vi "TOOLweb Zeit-Datum-Strings nach Zeitstempel.vi"(2 "Format":T1(ring), 3 "Zeit/Datum-String":string) -> (0 "Zeit-Cluster":T2, 1 "Zeitstempel":timestamp)   [LabVIEW 2020, in "FT-IR.lvlib" / "TOOLweb Interface.lvlib" / "TOOLweb Interface Hilfs-VIs.lvlib"]
doc: "Formt den TOOLweb-Zeit/Datum-String in einen Zeitstempel um. Der Ausgang \"Zeit-Cluster\" bietet einen einfachen Zugriff auf die einzelnen Elemente der Zeit/Datums-Information."
uses:
  TOOLweb Interface Hilfs-VIs.lvlib
  <vilib>/Utility/miscctls.llb/LVDateTimeRec.ctl
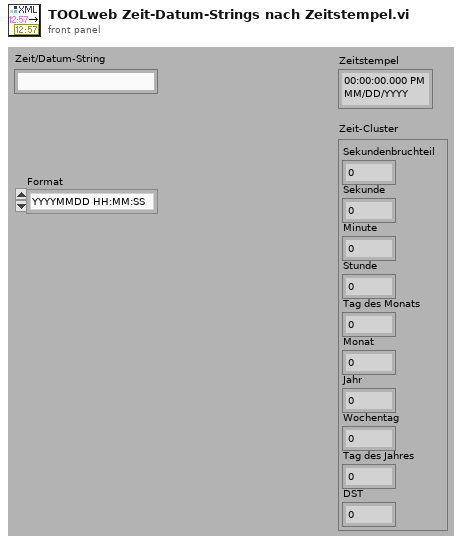
[diagram p1: front panel]
types:
  T1 = enum16{"YYYYMMDD HH:MM:SS", "[YYMMDD][HH:MM:SS]"}
  T2 = typedef "LVDateTimeRec.ctl" = cluster{"fractional second":dbl, "second":i32, "minute":i32, "hour":i32, "day of month":i32, "month":i32, "year":i32, "day of week":i32, "day of year":i32, "DST":i32}
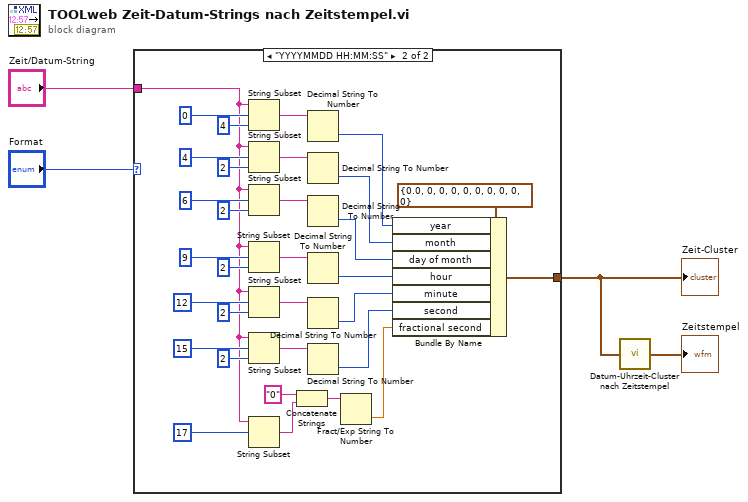
[diagram p0: block diagram]
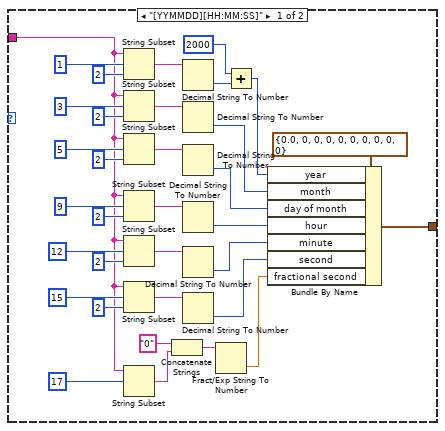
[diagram p2: hidden frame]
diagram:
  n1 = case shown="\"YYYYMMDD HH:MM:SS\"" "Format" {
    tunnel: [w37 w69] -> w4
    tunnel: "Zeit/Datum-String" -> [w8 w39]
    frame "[YYMMDD][HH:MM:SS]" {
      n2 = String Subset(string=w8, offset (0)=1 ("Offset (0)"), length (rest)=2 ("Länge (Rest)")) -> (substring=w24:string)
      n3 = String Subset(string=w8, offset (0)=3 ("Offset (0)"), length (rest)=2 ("Länge (Rest)")) -> (substring=w23:string)
      n4 = String Subset(string=w8, offset (0)=5 ("Offset (0)"), length (rest)=2 ("Länge (Rest)")) -> (substring=w22:string)
      n5 = String Subset(string=w8, offset (0)=9 ("Offset (0)"), length (rest)=2 ("Länge (Rest)")) -> (substring=w21:string)
      n6 = String Subset(string=w8, offset (0)=12 ("Offset (0)"), length (rest)=2 ("Länge (Rest)")) -> (substring=w20:string)
      n7 = String Subset(string=w8, offset (0)=15 ("Offset (0)"), length (rest)=2 ("Länge (Rest)")) -> (substring=w19:string)
      n8 = String Subset(string=w8, offset (0)=17 ("Offset (0)")) -> (substring=w11:string)  [unwired: 1 out]
      n9 = Concatenate Strings("0" ("String"), w11) -> (w10:string)
      n10 = Decimal String To Number(string=w24) -> (number=w7:i32)  [unwired: 3 out]
      n11 = Decimal String To Number(string=w23) -> (number=w18:i32)  [unwired: 3 out]
      n12 = Decimal String To Number(string=w22) -> (number=w17:i32)  [unwired: 3 out]
      n13 = Decimal String To Number(string=w21) -> (number=w16:i32)  [unwired: 3 out]
      n14 = Decimal String To Number(string=w20) -> (number=w15:i32)  [unwired: 3 out]
      n15 = Decimal String To Number(string=w19) -> (number=w14:i32)  [unwired: 3 out]
      n16 = Fract/Exp String To Number(string=w10) -> (number=w9:dbl)  [unwired: 4 out]
      n17 = Add(x=2000, y=w7) -> (x+y=w6:i32)
      n18 = Bundle By Name(cluster=T2 {"fractional second"=0.0, "second"=0, "minute"=0, "hour"=0, "day of month"=0, "month"=0, "year"=0, "day of week"=0, "day of year"=0, "DST"=0} ("Datum/Zeit"), "year"=w6, "month"=w18, "day of month"=w17, "hour"=w16, "minute"=w15, "second"=w14, "fractional second"=w9) -> (w37:T2)
    }
    frame "YYYYMMDD HH:MM:SS" {
      n19 = String Subset(string=w39, offset (0)=0 ("Offset (0)"), length (rest)=4 ("Länge (Rest)")) -> (substring=w56:string)
      n20 = String Subset(string=w39, offset (0)=4 ("Offset (0)"), length (rest)=2 ("Länge (Rest)")) -> (substring=w55:string)
      n21 = String Subset(string=w39, offset (0)=6 ("Offset (0)"), length (rest)=2 ("Länge (Rest)")) -> (substring=w54:string)
      n22 = String Subset(string=w39, offset (0)=9 ("Offset (0)"), length (rest)=2 ("Länge (Rest)")) -> (substring=w53:string)
      n23 = String Subset(string=w39, offset (0)=12 ("Offset (0)"), length (rest)=2 ("Länge (Rest)")) -> (substring=w52:string)
      n24 = String Subset(string=w39, offset (0)=15 ("Offset (0)"), length (rest)=2 ("Länge (Rest)")) -> (substring=w51:string)
      n25 = String Subset(string=w39, offset (0)=17 ("Offset (0)")) -> (substring=w42:string)  [unwired: 1 out]
      n26 = Concatenate Strings("0" ("String"), w42) -> (w41:string)
      n27 = Decimal String To Number(string=w56) -> (number=w50:i32)  [unwired: 3 out]
      n28 = Decimal String To Number(string=w55) -> (number=w49:i32)  [unwired: 3 out]
      n29 = Decimal String To Number(string=w54) -> (number=w48:i32)  [unwired: 3 out]
      n30 = Decimal String To Number(string=w53) -> (number=w47:i32)  [unwired: 3 out]
      n31 = Decimal String To Number(string=w52) -> (number=w46:i32)  [unwired: 3 out]
      n32 = Decimal String To Number(string=w51) -> (number=w45:i32)  [unwired: 3 out]
      n33 = Fract/Exp String To Number(string=w41) -> (number=w40:dbl)  [unwired: 4 out]
      n34 = Bundle By Name(cluster=T2 {"fractional second"=0.0, "second"=0, "minute"=0, "hour"=0, "day of month"=0, "month"=0, "year"=0, "day of week"=0, "day of year"=0, "DST"=0} ("Datum/Zeit"), "year"=w50, "month"=w49, "day of month"=w48, "hour"=w47, "minute"=w46, "second"=w45, "fractional second"=w40) -> (w69:T2)
    }
  }
  "Zeit-Cluster" <- w4
  n35 = call "Datum-Uhrzeit-Cluster nach Zeitstempel.vi"("Datum/Zeit"=w4) -> ("Zeitstempel"=→"Zeitstempel":timestamp)
